vi "oa_RMS Average (1 Channel).vi"(6 "averaging parameters":T2={"averaging mode"=enum."No averaging", "weighting mode"=enum."Exponential", "number of averages"=10, "linear mode"=enum."One shot"} {"number of averages" min=1 step=1}, 7 "processing control in":T1(ring), 8 "error in (no error)":errorcluster, 11 "Y":dbl[][](array[numeric]) format="%.2f") -> (0 "error out":errorcluster, 1 "averages completed":dbl, 2 "averaging done":bool, 3 "Y out":dbl[](array[numeric]) format="%.2f")   [LabVIEW 2017, in "SoundVib_Resampling.lvlib"]
uses:
  <vilib>/addons/Sound and Vibration/Order Analysis/Resample Order Tracking/SoundVib_Resampling.lvlib
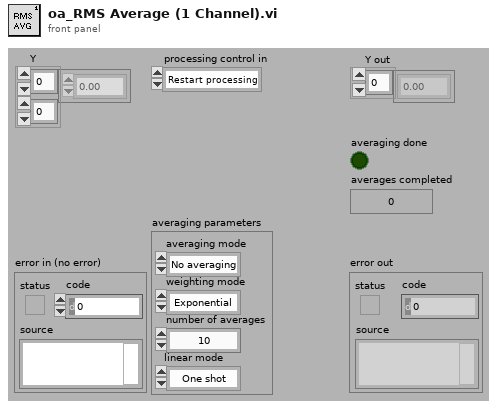
[diagram p1: front panel]
types:
  T1 = enum16{"Restart processing", "Continue processing", "Skip processing"}
  T2 = cluster{"averaging mode":enum16{"No averaging", "Vector averaging", "RMS averaging", "Peak hold"}, "weighting mode":enum16{"Linear", "Exponential"}, "number of averages":u32, "linear mode":enum16{"One shot", "Auto restart"}}
  T3 = cluster{"complex FFT":cdb[], "power spectrum":dbl[], "averages completed":dbl}
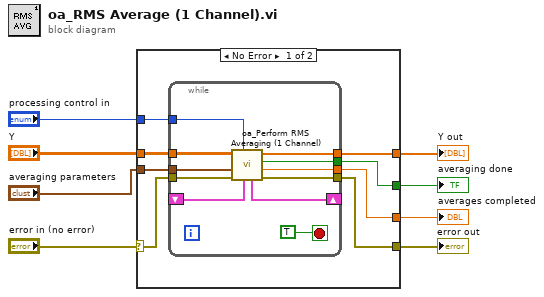
[diagram p0: block diagram]
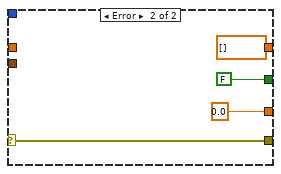
[diagram p2: hidden frame]
diagram:
  n1 = case shown="No Error" "error in (no error)" {
    selector: "error in (no error)" -> [w13 w31]
    tunnel: [w12 w31] -> w2
    tunnel: "Y" -> [w16 _]
    tunnel: "processing control in" -> [w15 _]
    tunnel: "averaging parameters" -> [w14 _]
    tunnel: [w11 dbl[] [] ("Y out")] -> w1
    tunnel: [w10 FALSE ("averaging done")] -> w4
    tunnel: [w9 0.0 ("averages completed")] -> w3
    frame No Error {
      n2 = while {
        tunnel: w16 -> [w27]
        tunnel: w15 -> [w26]
        tunnel: w14 -> [w25]
        tunnel: w13 -> [w24]
        tunnel: [w23] -> w12
        tunnel: [w22] -> w11
        tunnel: [w21] -> w10
        tunnel: [w20] -> w9
        shift-right: [w19] -> _
        shift-left: _ -> [w18]
        stop <- TRUE stop-if-true
        n3 = call <vilib>:"oa_Perform RMS Averaging (1 Channel).vi"("averaging state info in"=w18, "processing control in"=w26, "error in (no error)"=w24, "averaging parameters"=w25, "Y"=w27) -> ("error out"=w23:errorcluster, "averages completed"=w20:dbl, "averaging done"=w21:bool, "Y out"=w22:dbl[], "averaging state info out"=w19:T3)  [unwired: 2 in]
      }
    }
    frame Error {
    }
  }
  "averaging done" <- w4
  "averages completed" <- w3
  "Y out" <- w1
  "error out" <- w2
